vi "Frequency Response Reference to Frequency.vi"(9 "reference frequency":dbl, 10 "frequency":dbl[](array[numeric]), 11 "amplitude (dBPL)":dbl[](array[numeric])) -> (3 "amplitude (dBr)":dbl[](array[numeric]))   [LabVIEW 2022 SP3]
uses:
  <vilib>/Analysis/1siggen.llb/Ramp Pattern by Samples.vi
  <vilib>/gmath/NI_Gmath.lvlib
  <vilib>/Analysis/NI_AALBase.lvlib
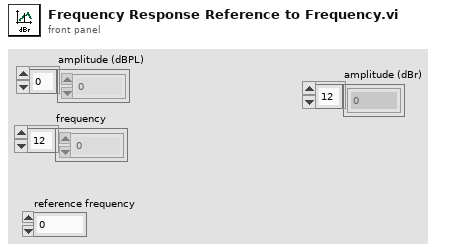
[diagram p1: front panel]
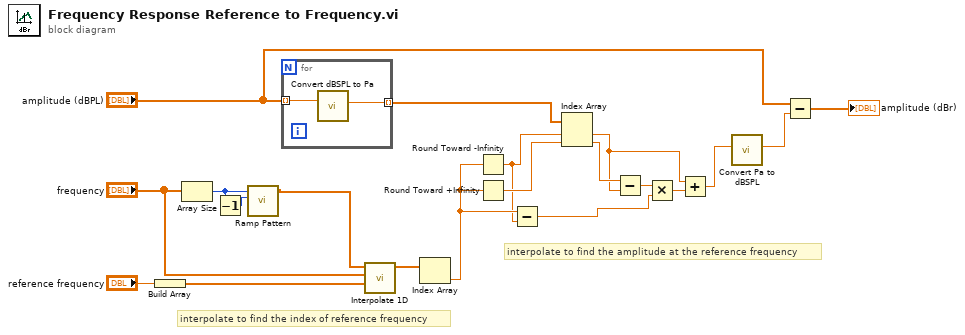
[diagram p0: block diagram]
diagram:
  # "interpolate to find the amplitude at the reference frequency"
  # "interpolate to find the index of reference frequency"
  n1 = Build Array("reference frequency") -> (w19:dbl[])
  n2 = Array Size(array="frequency") -> (size(s)=w16:i32)
  n3 = Decrement(x=w16) -> (x-1=w15:i32)
  n4 = call-poly <vilib>:"Ramp Pattern.vi"("end"=w15, "samples"=w16) -> ("Ramp Pattern"=w17:dbl[])  [unwired: 8 in, 1 out]
  n5 = for {
    tunnel: "amplitude (dBPL)" -> [w22] mode=indexing
    tunnel: [w21] -> w5 mode=indexing
    n6 = call "Convert dBSPL to Pa.vi"("dB SPL"=w22) -> ("Pa rms"=w21:dbl)  [unwired: 9 in, 1 out]
  }
  n7 = call <vilib>:"Interpolate 1D.vi"("xi"=w19, "X"="frequency", "Y"=w17) -> ("yi"=w13:dbl[])  [unwired: 6 in, 2 out]
  n8 = Index Array(array=w13) -> (element=w12:dbl)  [unwired: 1 in]
  n9 = Round Toward -Infinity(1:w12) -> (0:w11:dbl)
  n10 = Round Toward +Infinity(x=w12) -> (ceil(x): smallest int >= x=w14:dbl)
  n11 = Subtract(x=w12, y=w11) -> (x-y=w8:dbl)
  n12 = Index Array(array=w5, index #1=w11, index #2=w14) -> (element #1=w6:dbl, element #2=w10:dbl)
  n13 = Subtract(x=w10, y=w6) -> (x-y=w9:dbl)
  n14 = Multiply(x=w9, y=w8) -> (x*y=w7:dbl)
  n15 = Add(x=w6, y=w7) -> (x+y=w4:dbl)
  n16 = call "Convert Pa to dBSPL.vi"("Pa rms"=w4) -> ("dBSPL"=w2:dbl)  [unwired: 10 in]
  n17 = Subtract(x="amplitude (dBPL)", y=w2) -> (x-y=→"amplitude (dBr)":dbl[])
